vi "Right Click.vi"(7 "object refs":T2, 8 "error in (no error)":errorcluster, 9 "Coords":T1, 10 "Event data":variant, 11 "Multi Column Listbox in":refnum<class "Multi Column Listbox.lvclass">) -> (0 "error out":errorcluster, 3 "Multi Column Listbox out":refnum<class "Multi Column Listbox.lvclass">)   [LabVIEW 2013, in "Table Manager.lvlib" / "Multi Column Listbox.lvclass"]
uses:
  Multi Column Listbox.lvclass
  TagSelectModule/Source/editor node/object ref.ctl
  <vilib>/NI/Tag Bus Data Framework/Configuration Editor/Classes/Engine Parent/Engine Parent Editor Node.lvclass
  <vilib>/NI/Tag Bus Data Framework/Configuration Editor/Classes/Module editor node/module editor node.lvclass
  <vilib>/Utility/miscctls.llb/LVPoint32TypeDef.ctl
  Multi Column Listbox.lvclass/Multi Column Listbox.ctl
  Table Manager/Table Manager.lvclass/Table Manager.ctl
  <vilib>/NI/Tag Bus Module Framework/module configuration/TBM module configuration.lvclass
  <vilib>/NI/Tag Bus/tag/tag descriptor.lvclass/tag descriptor.ctl
  Table Manager/Read ATM.vi
  <vilib>/NI/Tag Bus/tag/read tag name.vi
  <vilib>/NI/Tag Bus Data Framework/Configuration Editor/Classes/Module editor node/Read Module Configuration.vi
  <vilib>/NI/Tag Bus/tag/tag descriptor.lvclass
  TagSelectModule/Source/editor node/tag select module editor node.lvclass
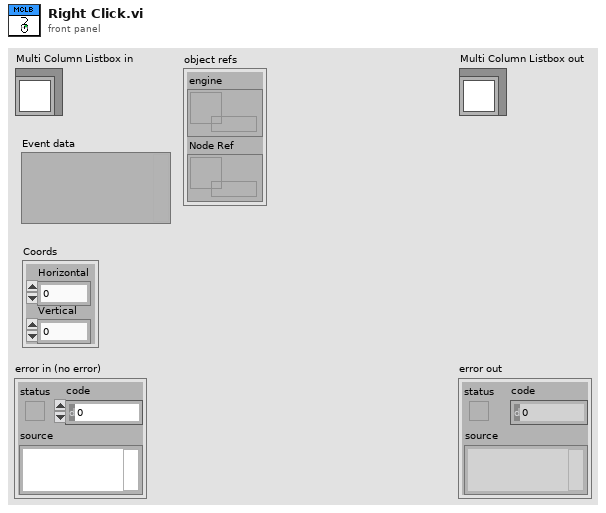
[diagram p1: front panel]
types:
  T1 = typedef "LVPoint32TypeDef.ctl" = cluster{"Horizontal":i32, "Vertical":i32}
  T2 = typedef "tag select module editor node.lvclass/object ref.ctl" = cluster{"engine":refnum<data-value>, "Node Ref":refnum<data-value>}
  T3 = typedef "LVRowAndColumnTypeDef.ctl" = cluster{"Row":i32, "Column":i32}
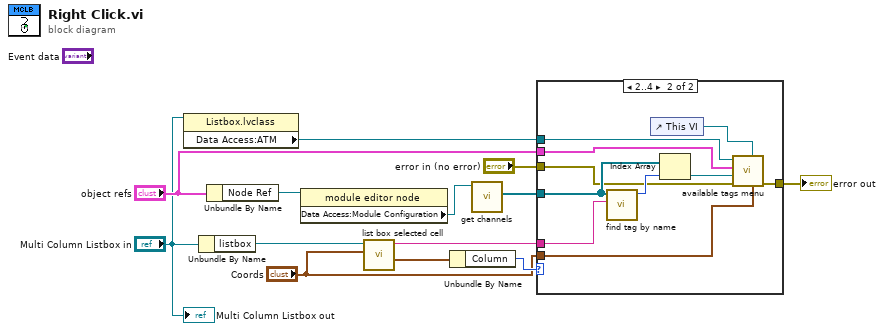
[diagram p0: block diagram]
diagram:
  n1 = property class="Listbox.lvclass"(reference="Multi Column Listbox in") -> ("Data Access:ATM"=w1:refnum<user-event>)  [unwired: 1 in, 2 out]
  n2 = Unbundle By Name("Multi Column Listbox in") -> ("listbox"=w7:refnum<vi>)
  n3 = Unbundle By Name("object refs") -> ("Node Ref"=w8:refnum<data-value>)
  n4 = property class="module editor node"(reference=w8) -> ("Data Access:Module Configuration"=w13:refnum<class "TBM module configuration.lvclass">)  [unwired: 1 in, 2 out]
  n5 = call "list box selected cell.vi"("Coords"="Coords", "MulticolumnListbox in"=w7) -> ("cell position"=w10:T3, "tag select name"=w11:string)  [unwired: 6 in, 2 out]
  n6 = Unbundle By Name(w10) -> ("Column"=w9:i32)
  n7 = call-dynamic "get channels.vi"("module configuration in"=w13) -> ("channels"=w12:refnum<class "TBM channel.lvclass">[])  [unwired: 9 in, 1 out]
  n8 = case shown="2..4" w9 {
    tunnel: w12 -> [_ w23]
    tunnel: w11 -> [_ w22]
    tunnel: "Coords" -> [_ w18]
    tunnel: w1 -> [_ w19]
    tunnel: "object refs" -> [_ w17]
    tunnel: [w14 w16] -> w4
    tunnel: "error in (no error)" -> [w14 w15]
    frame 0, Default {
    }
    frame 2..4 {
      n9 = call <vilib>:"find tag by name.vi"("name"=w22, "tags in"=w23) -> ("index"=w24:i32)  [unwired: 9 in]
      n10 = control-ref of="This VI"() -> (w21:refnum<vi>)
      n11 = Index Array(array=w23, index=w24) -> (element=w20:refnum<class "TBM channel.lvclass">)
      n12 = call "available tags menu.vi"("Point32"=w18, "parent vi reference"=w21, "error in"=w15, "channel to map to"=w20, "object ref"=w17, "ATM"=w19) -> ("error out"=w16:errorcluster)  [unwired: 5 in]
    }
  }
  "error out" <- w4
  "Multi Column Listbox out" <- "Multi Column Listbox in"
